vi "Library Name.vi"() -> (3 "library name":string)   [LabVIEW 2023, in "UDPlog.lvlib" / "UDPlog Transceiver.lvclass"]
uses:
  UDPlog Transceiver.lvclass
  UDPlog Transceiver.lvclass/UDPlog Transceiver.ctl
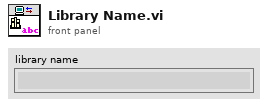
[diagram p1: front panel]
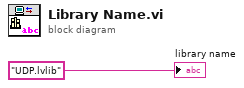
[diagram p0: block diagram]
diagram:
  "library name" <- "UDP.lvlib" ("base error code")
